vi "Parse Test Results.vi"(11 "Raw Test Results":string) -> (2 "Test Suites":T1[](array[typedef]), 3 "Test Header":T3={"name"="", "tests"=-1, "failures"=-1, "errors"=-1, "time"=-1.0, "disabled"=-1, "skipped"=-1, "skips"=-1, "timestamp"=-1.0, "hostname"="", "id"="", "package"="", "assertions"=-1, "file"="", "skip"="", "log"="", "url"=""})   [LabVIEW 2014, in "VI Tester Parsing.lvlib"]
uses:
  VI Tester Parsing.lvlib
  <vilib>/ni/JUnit Results API/Controls/Test Suite Attribute Values.ctl
  Test Suite.ctl
  Test Case.ctl
  <vilib>/ni/JUnit Results API/JUnit API.lvlib
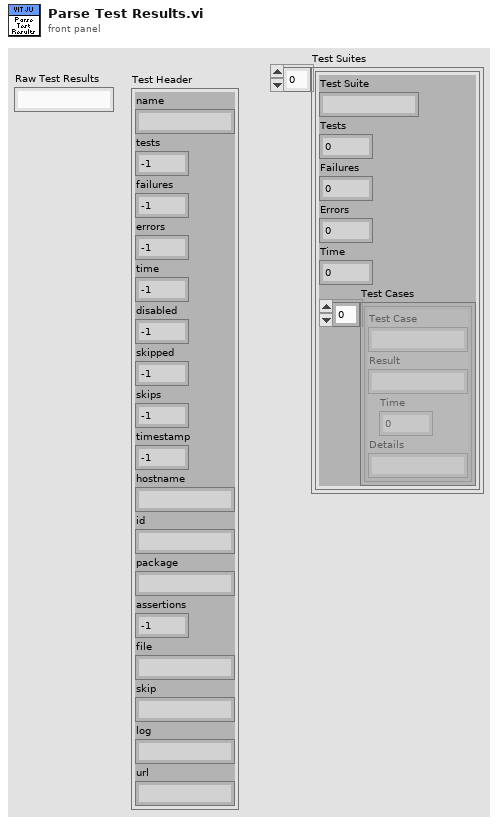
[diagram p1: front panel]
types:
  T1 = typedef "VI Tester Parsing.lvlib/Test Suite.ctl" = cluster{"Test Suite":string, "Tests":i32, "Failures":i32, "Errors":i32, "Time":dbl, "Test Cases":T2[]}
  T2 = typedef "VI Tester Parsing.lvlib/Test Case.ctl" = cluster{"Test Case":string, "Result":string, "Time":dbl, "Details":string}
  T3 = typedef "JUnit API.lvlib/Test Suite Attribute Values.ctl" = cluster{"name":string, "tests":i32, "failures":i32, "errors":i32, "time":dbl, "disabled":i32, "skipped":i32, "skips":i32, "timestamp":dbl, "hostname":string, "id":string, "package":string, "assertions":i32, "file":string, "skip":string, "log":string, "url":string}
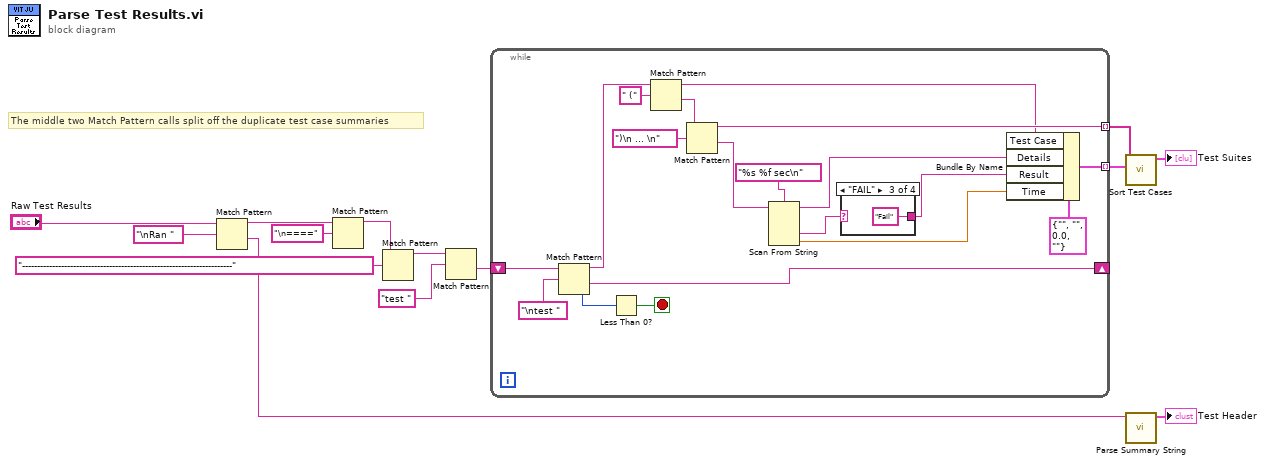
[diagram p0: block diagram]
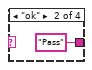
[diagram p3: hidden frame]
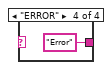
[diagram p4: hidden frame]
diagram:
  # "The middle two Match Pattern calls split off the duplicate test case summaries"
  n1 = Match Pattern(string="Raw Test Results", regular expression="\nRan ") -> (before substring=w6:string, after substring=w5:string)  [unwired: 1 in, 2 out]
  n2 = Match Pattern(string=w6, regular expression="\n====") -> (before substring=w10:string)  [unwired: 1 in, 3 out]
  n3 = Match Pattern(string=w10, regular expression="----------------------------------------------------------------------") -> (before substring=w12:string)  [unwired: 1 in, 3 out]
  n4 = Match Pattern(string=w12, regular expression="test " ("format string")) -> (after substring=w13:string)  [unwired: 1 in, 3 out]
  n5 = while {
    shift-right: [w30] -> _
    shift-left: w13 -> [w33]
    tunnel: [w28] -> w2 mode=indexing
    tunnel: [w21] -> w3 mode=indexing
    stop <- w31 stop-if-true
    n6 = Match Pattern(string=w33, regular expression="\ntest " ("format string")) -> (before substring=w23:string, after substring=w30:string, offset past match=w32:i32)  [unwired: 1 in, 1 out]
    n7 = Less Than 0?(x=w32) -> (x < 0?=w31:bool)
    n8 = Match Pattern(string=w23, regular expression=" (") -> (before substring=w19:string, after substring=w26:string)  [unwired: 1 in, 2 out]
    n9 = Match Pattern(string=w26, regular expression=")\n ... \n") -> (before substring=w21:string, after substring=w22:string)  [unwired: 1 in, 2 out]
    n10 = Scan From String(format string="%s %f sec\n", input string=w22) -> (remaining string=w16:string, output 1=w18:string, output 2=w17:dbl)  [unwired: 4 in, 2 out]
    n11 = case shown="\"FAIL\"" w18 {
      selector: w18 -> [w34 _ _ _]
      tunnel: [w34 "Pass" "Fail" "Error"] -> w15
      frame Default {
      }
      frame "ok" {
      }
      frame "FAIL" {
      }
      frame "ERROR" {
      }
    }
    n12 = Bundle By Name(cluster=T2 {"Test Case"="", "Result"="", "Time"=0.0, "Details"=""}, "Test Case"=w19, "Details"=w16, "Result"=w15, "Time"=w17) -> (w28:T2)
  }
  n13 = call "Sort Test Cases.vi"("Test Cases"=w2, "Test Suites"=w3) -> ("Test Suites"=→"Test Suites":T1[])  [unwired: 9 in]
  n14 = call "Parse Summary String.vi"("Summary String"=w5) -> ("Test Header"=→"Test Header":T3)  [unwired: 10 in]
